vi "Add HTTP Content.vi"(6 "ContentType":T1, 8 "error in (no error)":errorcluster, 10 "HttpContent To Add":refnum<class "HttpContent.lvclass">, 11 "HttpContent_Multipart in":refnum<class "HttpContent_Multipart.lvclass">) -> (0 "error out":errorcluster, 3 "HttpContent_Multipart out":refnum<class "HttpContent_Multipart.lvclass">)   [LabVIEW 2018, in "HttpClient_NET.lvlib" / "HttpContent_Multipart.lvclass"]
doc: "<b> </b> <b> </b>\nHttpClient_NET\nJustin Young - Viviota\nCopyright (c) 2021\nLicense: BSD"
uses:
  HttpContent_Multipart.lvclass
  C:/Viviota/Projects/R&D/__OpenSource/VIV_HTTP_REST_NET/HttpContent/HttpContent.lvclass
  Types/ContentType.ctl
  HttpContent/HttpContent.lvclass
  HttpContent/HttpContent.lvclass/HttpContent.ctl
  Read NET_MultipartContent.vi
  HttpContent/Accessors/Read NET_HttpContent.vi
  System.Net.Http
  HttpHeaders_content/HttpHeaders_Content.lvclass
  HttpClient_NET.lvlib
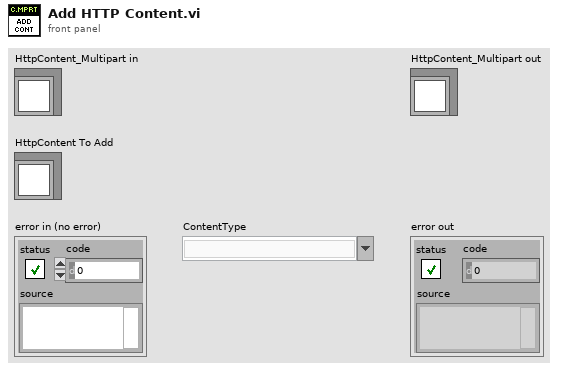
[diagram p1: front panel]
types:
  T1 = typedef "HttpClient_NET.lvlib/ContentType.ctl" = string
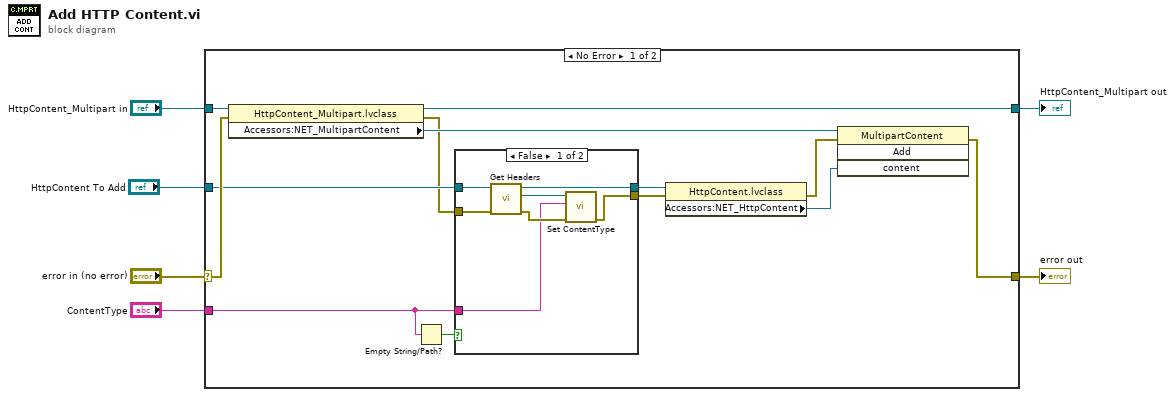
[diagram p0: block diagram]
diagram:
  n1 = case shown="No Error" "error in (no error)" {
    selector: "error in (no error)" -> [w19 w30]
    tunnel: [w7 w30] -> w5
    tunnel: [w17 w29] -> w3
    tunnel: "HttpContent_Multipart in" -> [w18 w29]
    tunnel: "HttpContent To Add" -> [w15 _]
    tunnel: "ContentType" -> [w10 _]
    frame No Error {
      n2 = property class="HttpContent_Multipart.lvclass"(reference=w18, error in=w19) -> (reference out=w17:refnum<class "HttpContent_Multipart.lvclass">, error out=w14:errorcluster, "Accessors:NET_MultipartContent"=w16:refnum<k24>)
      n3 = Empty String/Path?(string/path=w10) -> (empty?=w11:bool)
      n4 = case shown="False" w11 {
        tunnel: w15 -> [w26 w28]
        tunnel: w14 -> [w25 w27]
        tunnel: w10 -> [w22 _]
        tunnel: [w21 w27] -> w13
        tunnel: [w20 w28] -> w12
        frame False {
          n5 = call "Get Headers.vi"("error in (no error)"=w25, "HttpContent in"=w26) -> ("error out"=w24:errorcluster, "HTTPHeaders"=w23:refnum<class "HttpHeaders_Content.lvclass">, "HttpContent out"=w20:refnum<class "HttpContent.lvclass">)  [unwired: 7 in]
          n6 = call "Set ContentType.vi"("error in (no error)"=w24, "ContentType"=w22, "HttpHeaders_Content in"=w23) -> ("error out"=w21:errorcluster)  [unwired: 7 in, 1 out]
        }
        frame True {
        }
      }
      n7 = property class="HttpContent.lvclass"(reference=w12, error in=w13) -> (error out=w9:errorcluster, "Accessors:NET_HttpContent"=w8:refnum<k24>)  [unwired: 1 out]
      n8 = invoke class="MultipartContent" method="Add"(reference=w16, error in=w9, "content"=w8) -> (error out=w7:errorcluster)  [unwired: 1 in, 3 out]
    }
    frame Error {
    }
  }
  "error out" <- w5
  "HttpContent_Multipart out" <- w3
